vi "Open File.vi"() -> (2 "Angle":dbl[][](array[numeric]), 3 "Position":dbl[][](array[numeric]))   [LabVIEW 2020]
panel:
  out "data 2":string
  out "new file path 2":path
  out "data":string
  out "new file path":path
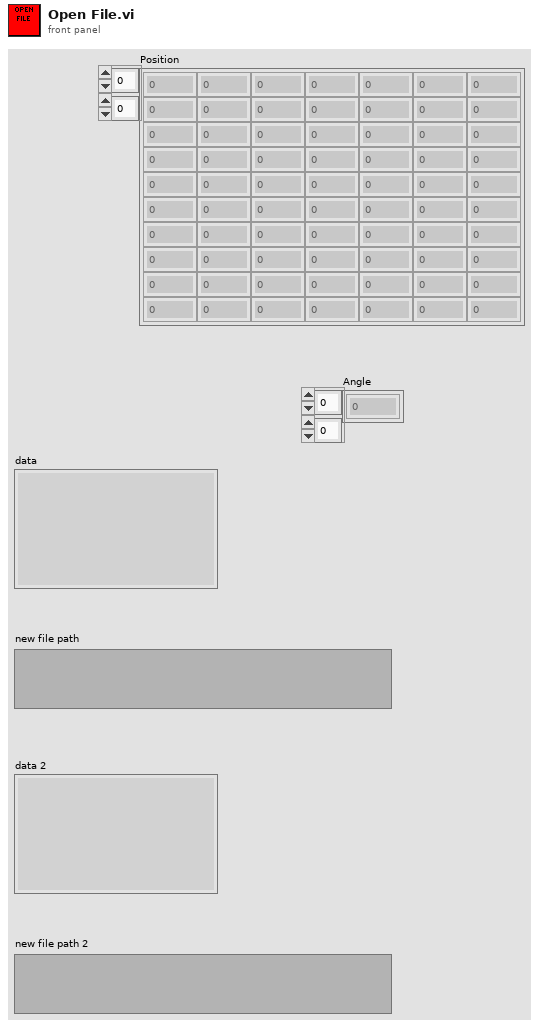
[diagram p1: front panel]
types:
  T1 = enum16{"open", "open or create", "create or replace", "create", "open (read only)"}
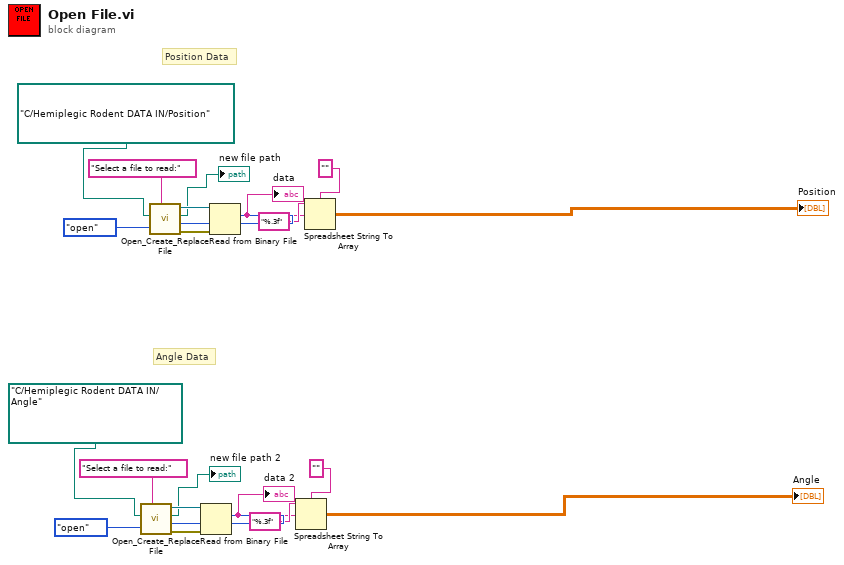
[diagram p0: block diagram]
diagram:
  # "Angle Data"
  # "Position Data"
  n1 = call <vilib>:"Open_Create_Replace File.vi"("prompt"="Select a file to read:", "function (open:0)"=T1."open", "start path  (Not A Path)"=path "C:/Hemiplegic Rodent DATA IN/Angle") -> ("error out"=w6:errorcluster, "file size (bytes)"=w11:i32, "new file path"=→"new file path 2":path, "refnum"=w10:refnum<file>)  [unwired: 5 in]
  n2 = call <vilib>:"Open_Create_Replace File.vi"("prompt"="Select a file to read:", "function (open:0)"=T1."open", "start path  (Not A Path)"=path "C:/Hemiplegic Rodent DATA IN/Position") -> ("error out"=w16:errorcluster, "file size (bytes)"=w21:i32, "new file path"=→"new file path":path, "refnum"=w20:refnum<file>)  [unwired: 5 in]
  n3 = Read from Binary File ("Read File")(8:w6, 10:w11, 11:w10) -> (2:w3:string)  [unwired: 3 in, 3 out]
  "data 2" <- w3
  n4 = Read from Binary File ("Read File")(8:w16, 10:w21, 11:w20) -> (2:w13:string)  [unwired: 3 in, 3 out]
  "data" <- w13
  n5 = Spreadsheet String To Array(delimiter (Tab)="", format string="%.3f" ("String"), spreadsheet string=w3) -> (array=→"Angle":dbl[][])  [unwired: 1 in]
  n6 = Spreadsheet String To Array(delimiter (Tab)="", format string="%.3f" ("String"), spreadsheet string=w13) -> (array=→"Position":dbl[][])  [unwired: 1 in]
